vi "flatten (bool 2d).vi"(3 "array":bool[][](array[boolean])) -> (1 "flattened":bool[](array[boolean]))   [LabVIEW 2012, in "common.lvlib"]
uses:
  common.lvlib
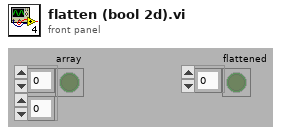
[diagram p1: front panel]
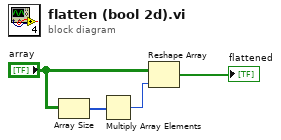
[diagram p0: block diagram]
diagram:
  n1 = Array Size(array="array") -> (size(s)=w4:i32[])
  n2 = Multiply Array Elements(1:w4) -> (0:w2:i32)
  n3 = Reshape Array("array", w2) -> (→"flattened":bool[])
